vi "DAQ_DECM Close.vi"(0 "DAQmx Tasks":T1, 11 "error in":errorcluster) -> (15 "error out":errorcluster)   [LabVIEW 2021, in "DAQ_Digital Edge Count Measurement.lvlib"]
doc: "Aborts and clears the tasks used in Digital Edge Count Measurement."
uses:
  DAQ_Digital Edge Count Measurement.lvlib
  Typedefs/DAQmx Tasks.ctl
panel:
  # "Inputs"
  # "Outputs"
  # "Overview:\nThis VI closes the Digital Edge Count Measurement DAQmx Task.\n\nHardware Requirement: A compatible PXI, PCIe, USB, cDAQ or Testscale device \n\nSoftware Requirement: NI DAQmx 2022Q4 or later\n\nInstructions:\n1. Input the digital edge count measurement task through DAQmx Tasks control.\n2. This VI aborts and clears the Digital Edge Count Measurement task."
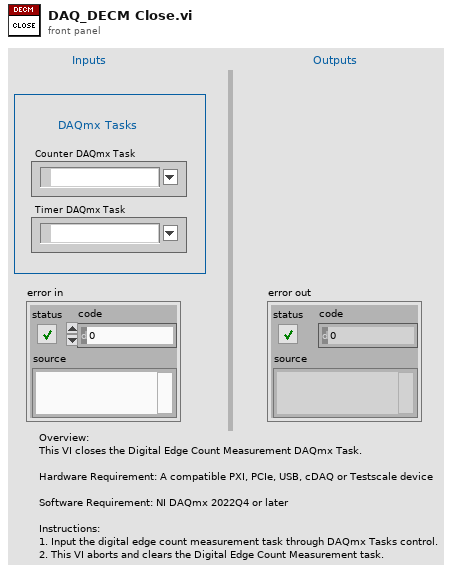
[diagram p1: front panel]
types:
  T1 = typedef "DAQ_Digital Edge Count Measurement.lvlib/DAQmx Tasks.ctl" = cluster{"Counter DAQmx Task":refnum<k21>, "Timer DAQmx Task":refnum<k21>}
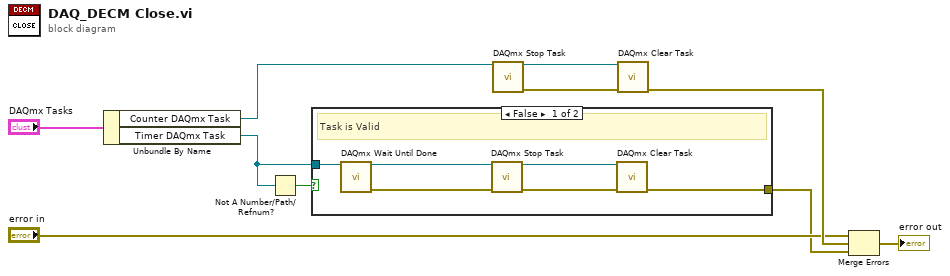
[diagram p0: block diagram]
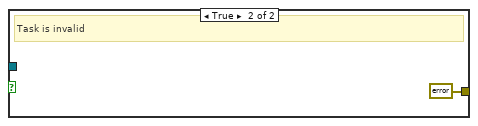
[diagram p2: hidden frame]
diagram:
  n1 = Unbundle By Name("DAQmx Tasks") -> ("Counter DAQmx Task"=w2:refnum<k21>, "Timer DAQmx Task"=w1:refnum<k21>)
  n2 = Not A Number/Path/Refnum?(number/path/refnum=w1) -> (NaN/Path/Refnum?=w4:bool)
  n3 = case shown="False" w4 {
    tunnel: [w13 errorcluster {"status"=FALSE, "code"=0, "source"=""} ("error out")] -> w5
    tunnel: w1 -> [w11 _]
    frame False {
      # "Task is Valid"
      n4 = call <vilib>:"DAQmx Wait Until Done.vi"("task/channels in"=w11) -> ("task out"=w15:refnum<k21>, "error out"=w14:errorcluster)  [unwired: 13 in]
      n5 = call <vilib>:"DAQmx Stop Task.vi"("task/channels in"=w15, "error in"=w14) -> ("task out"=w12:refnum<k21>, "error out"=w16:errorcluster)  [unwired: 12 in]
      n6 = call <vilib>:"DAQmx Clear Task.vi"("task in"=w12, "error in"=w16) -> ("error out"=w13:errorcluster)  [unwired: 13 in]
    }
    frame True {
      # "Task is invalid"
    }
  }
  n7 = call <vilib>:"DAQmx Stop Task.vi"("task/channels in"=w2) -> ("task out"=w10:refnum<k21>, "error out"=w9:errorcluster)  [unwired: 13 in]
  n8 = call <vilib>:"DAQmx Clear Task.vi"("task in"=w10, "error in"=w9) -> ("error out"=w7:errorcluster)  [unwired: 13 in]
  n9 = Merge Errors("error in", w7, w5) -> (→"error out":errorcluster)
